vi "Eval Formula String.vi"(2 "error in (no error)":errorcluster, 3 "formula":string) -> (0 "error out":errorcluster, 1 "y value":dbl format="%.2f")   [LabVIEW 2017, in "NI_Gmath.lvlib"]
doc: "Interprets a string as a numeric calculation and determines the result."
uses:
  <vilib>/gmath/NI_Gmath.lvlib
panel:
  # "Example:\n\n formula: sinh(6.3*sqrt(2.0))"
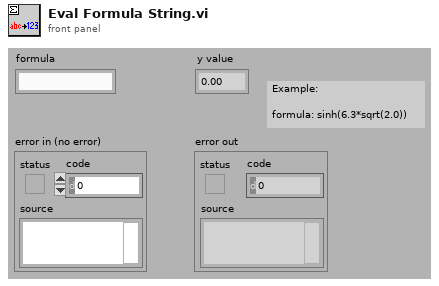
[diagram p1: front panel]
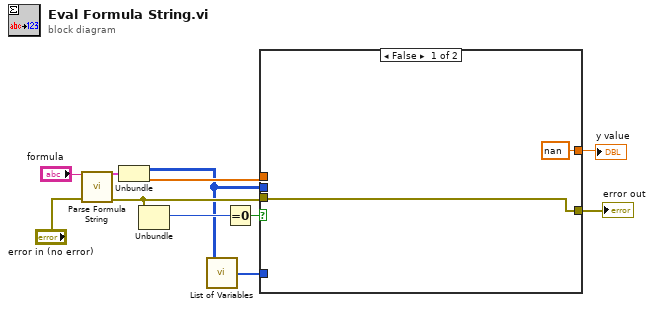
[diagram p0: block diagram]
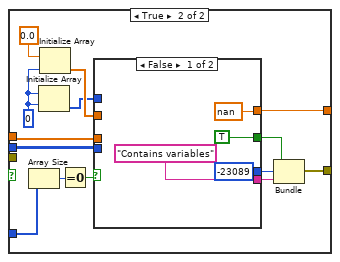
[diagram p2: hidden frame]
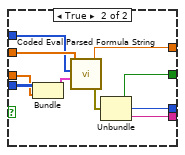
[diagram p3: hidden frame]
diagram:
  n1 = call <vilib>:"Parse Formula String.vi"("error in (no error)"="error in (no error)", "formula"="formula") -> ("error out"=w7:errorcluster, "Parsed Formula"=w5:cluster{"Table":i32[][], "Y Values":dbl[]})
  n2 = Unbundle(w5) -> ("Table"=w3:i32[][], "Y Values"=w4:dbl[])
  n3 = Unbundle(w7) -> ("code"=w6:i32)  [unwired: 2 out]
  n4 = call <vilib>:"List of Variables.vi"("Table"=w3) -> ("List of variables"=w8:i32[])
  n5 = Equal To 0?(x=w6) -> (x = 0?=w10:bool)
  n6 = case shown="False" w10 {
    tunnel: [nan w26] -> w9
    tunnel: w7 -> [w12 _]
    tunnel: w4 -> [_ w19]
    tunnel: w3 -> [_ w27]
    tunnel: w8 -> [_ w18]
    tunnel: [w12 w14] -> w1
    frame False {
    }
    frame True {
      w25 = 0
      n7 = Array Size(array=w18) -> (size(s)=w21:i32)
      n8 = Initialize Array(w25, w25) -> (w22:i32[])
      n9 = Initialize Array(0.0, w25) -> (w23:dbl[])
      n10 = Equal To 0?(x=w21) -> (x = 0?=w20:bool)
      n11 = case shown="False" w20 {
        tunnel: w22 -> [_ w35]
        tunnel: w23 -> [_ w36]
        tunnel: [-23089 w38] -> w16
        tunnel: [nan w41] -> w26
        tunnel: w27 -> [_ w33]
        tunnel: w19 -> [_ w32]
        tunnel: [TRUE w39] -> w17
        tunnel: ["Contains variables" w37] -> w15
        frame False {
        }
        frame True {
          n12 = Bundle("Table"=w33, "Y Values"=w32) -> (w34:cluster{"Table":i32[][], "Y Values":dbl[]})  [unwired: 1 in]
          n13 = call <vilib>:"Coded Eval Parsed Formula String.vi"("Parsed Formula"=w34, "Variables"=w35, "X Values"=w36) -> ("error out"=w40:errorcluster, "y value"=w41:dbl)  [unwired: 1 in]
          n14 = Unbundle(w40) -> ("status"=w39:bool, "code"=w38:i32, "source"=w37:string)
        }
      }
      n15 = Bundle("status"=w17, "code"=w16, "source"=w15) -> (w14:errorcluster)  [unwired: 1 in]
    }
  }
  "y value" <- w9
  "error out" <- w1
